vi "to_U16.vi"(8 "error_in":errorcluster, 10 "variable_start_index":i32, 11 "byte_array":u8[](array[numeric])) -> (0 "error_out":errorcluster, 3 "U16":u16)   [LabVIEW 2020]
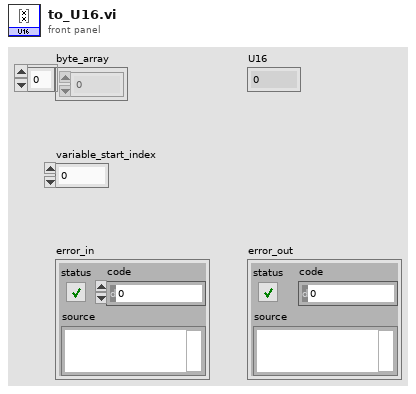
[diagram p1: front panel]
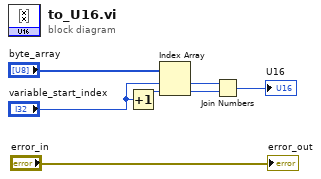
[diagram p0: block diagram]
diagram:
  n1 = Increment(x="variable_start_index") -> (x+1=w3:i32)
  n2 = Index Array(array="byte_array", index #1="variable_start_index", index #2=w3) -> (element #1=w6:u8, element #2=w7:u8)
  n3 = Join Numbers(hi=w6, lo=w7) -> ((hi.lo)=→"U16":u16)
  "error_out" <- "error_in"
